vi "FIU Global Strings.vi"() -> ()   [LabVIEW 2011, in "PXI-2510 Custom Device.lvlib"]
uses:
  PXI-2510 Custom Device.lvlib
panel:
  in  "Fault Bus Description":string="The Fault Bus has 6 different options: Default, Input 0, Input 1, Input 2, Input 3, and Main Bus Only.\n\nDefault: Does not make a call to the driver.\n\nInput 0,1,2,3: Close thier respective lines so that both the Main Bus and the Input Line is connected to the Fault Bus\n\nMain Bus Only: Disconnects Inputs 0,1,2, and 3 so that the Main Bus line is the only one connected to the Fault Bus"
  in  "Fault Channel Description":string="The \"Name (Alias)\" for each channel may be changed. The \"Hardware Channel #\" cannot be changed by the user, and represents the actual Fault Channel being controller.\n\nThe Fault Default Value sets the default state for the channel."
  in  "Fault Bus Input Selector":string="Fault Bus Input Selector"
  in  "Channel Fault":string="Channel Fault"
  in  "FIU Channel #":string="FIU Channel #"
  in  "Hardware Device Name":string="Hardware Device Name"
  in  "FIU Description":string="This is a Custom Device for the PXI-2510 FIU."
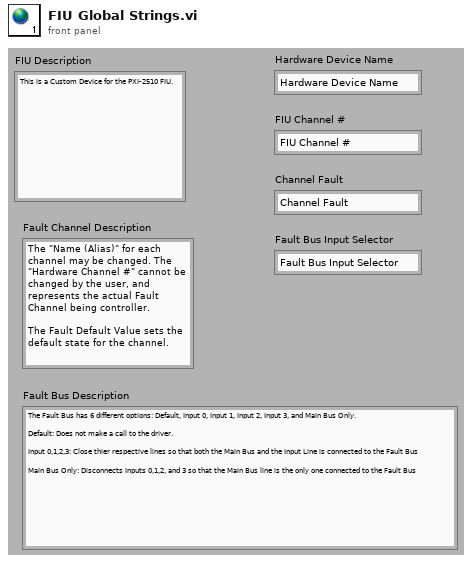
[diagram p1: front panel]
diagram:
